vi "Table Set Header Name and Data (String).vi"(9 "Data":string[][](array[string]), 10 "Header":string[](array[string]), 11 "Table Ref":refnum<vi>) -> ()   [LabVIEW 2023]
panel:
  out "Array":string[][](array[string])
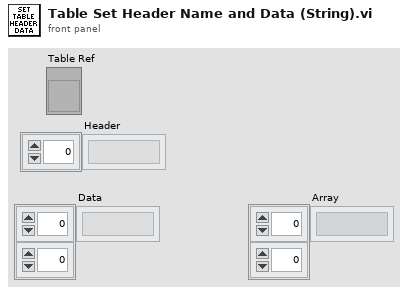
[diagram p1: front panel]
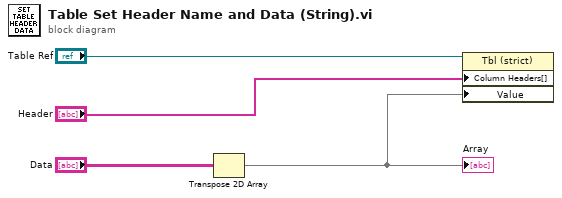
[diagram p0: block diagram]
diagram:
  n1 = Transpose 2D Array(2D array="Data") -> (transposed array=w1:string[][])
  "Array" <- w1
  n2 = property on="Property Node" class="Tbl (strict)"(reference="Table Ref", "Column Headers[]"="Header", "Value"=w1) -> ()  [unwired: 1 in, 2 out]
